vi "Clean_Delete_Selection.vi"(1 "Input Selection":i32[](array[numeric]), 2 "Input Sequence":cluster{string, string[], dbl[], dbl}[](array[cluster])) -> (0 "Output Selection":i32[](array[numeric]))   [LabVIEW 2011]
doc: "This VI will ensure that only one API command for a given ID in the Input Sequence is selected."
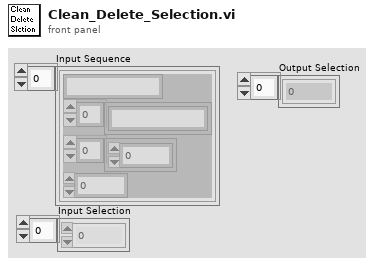
[diagram p1: front panel]
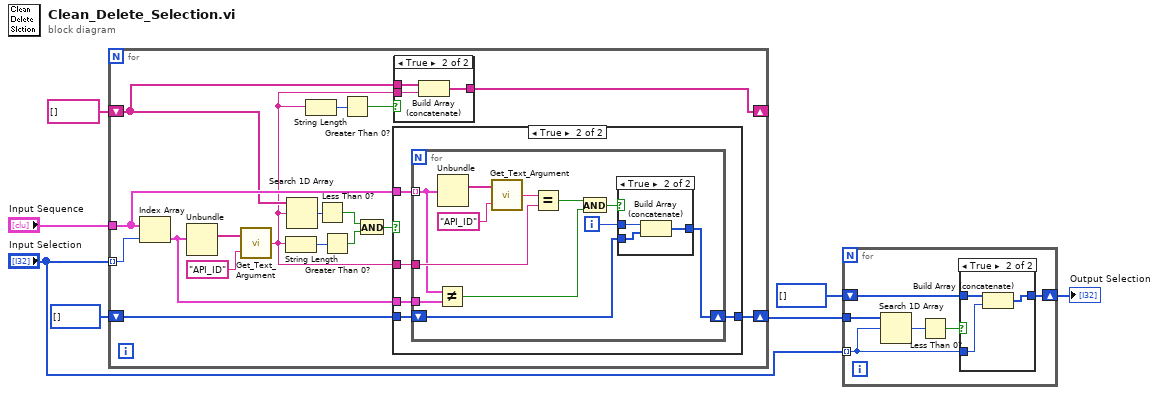
[diagram p0: block diagram]
diagram:
  n1 = for {
    tunnel: "Input Selection" -> [w21] mode=indexing
    tunnel: "Input Sequence" -> [w22]
    shift-right: [w20] -> w4
    shift-left: i32[] [] -> [w19]
    shift-right: [w17] -> _
    shift-left: string[] [] -> [w16]
    n2 = Index Array(array=w22, index=w21) -> (element=w8:cluster{string, string[], dbl[], dbl})
    n3 = Unbundle(w8) -> (w24:string[])  [unwired: 3 out]
    n4 = call "Get_Text_Argument.vi"("Argument"="API_ID", "Argument List"=w24) -> ("Text"=w10:string)
    n5 = String Length(string=w10) -> (length=w23:i32)
    n6 = Search 1D Array(1D array=w16, element=w10) -> (index of element=w15:i32)  [unwired: 1 in]
    n7 = String Length(string=w10) -> (length=w11:i32)
    n8 = Less Than 0?(x=w15) -> (x < 0?=w14:bool)
    n9 = Greater Than 0?(x=w23) -> (x > 0?=w12:bool)
    n10 = Greater Than 0?(x=w11) -> (x > 0?=w9:bool)
    n11 = And(x=w14, y=w12) -> (x .and. y?=w13:bool)
    n12 = case shown="True" w13 {
      tunnel: w22 -> [_ w34]
      tunnel: w10 -> [_ w33]
      tunnel: w19 -> [w29 w32]
      tunnel: [w29 w31] -> w20
      tunnel: w8 -> [_ w30]
      frame False {
      }
      frame True {
        n13 = for {
          tunnel: w34 -> [w35] mode=indexing
          tunnel: w33 -> [w43]
          shift-right: [w40] -> w31
          shift-left: w32 -> [w38]
          tunnel: w30 -> [w36]
          i -> [w39]
          n14 = Not Equal?(x=w35, y=w36) -> (x != y?=w41:bool)
          n15 = Unbundle(w35) -> (w45:string[])  [unwired: 3 out]
          n16 = call "Get_Text_Argument.vi"("Argument"="API_ID", "Argument List"=w45) -> ("Text"=w44:string)
          n17 = Equal?(x=w44, y=w43) -> (x = y?=w42:bool)
          n18 = And(x=w42, y=w41) -> (x .and. y?=w37:bool)
          n19 = case shown="True" w37 {
            tunnel: [w47 w50] -> w40
            tunnel: w39 -> [_ w49]
            tunnel: w38 -> [w47 w48]
            frame False {
            }
            frame True {
              n20 = Build Array (concatenate)(w49, w48) -> (w50:i32[])
            }
          }
        }
      }
    }
    n21 = case shown="True" w9 {
      tunnel: [w25 w28] -> w17
      tunnel: w16 -> [w25 w27]
      tunnel: w10 -> [_ w26]
      frame False {
      }
      frame True {
        n22 = Build Array (concatenate)(w27, w26) -> (w28:string[])
      }
    }
  }
  n23 = for {
    tunnel: "Input Selection" -> [w53] mode=indexing
    tunnel: w4 -> [w56]
    shift-right: [w51] -> w2
    shift-left: i32[] [] -> [w52]
    n24 = Search 1D Array(1D array=w56, element=w53) -> (index of element=w55:i32)  [unwired: 1 in]
    n25 = Less Than 0?(x=w55) -> (x < 0?=w54:bool)
    n26 = case shown="True" w54 {
      tunnel: w53 -> [_ w59]
      tunnel: w52 -> [w57 w60]
      tunnel: [w57 w58] -> w51
      frame False {
      }
      frame True {
        n27 = Build Array (concatenate)(w60, w59) -> (w58:i32[])
      }
    }
  }
  "Output Selection" <- w2
